vi "construct_response_generic.vi"(0 "command in":T3=enum."configure_rf", 1 "Status":T2, 5 "generic_info":string, 7 "datatype":T1, 9 "data in":variant, 11 "error in (no error) 2":errorcluster, 12 "source":string) -> (6 "Multipart message":string[](array[string]), 8 "Multipart message DVR out":refnum<data-value>, 14 "parameters JSON":string, 15 "error out 2":errorcluster)   [LabVIEW 2019, in "mmW_commands.lvlib"]
uses:
  mmW_commands.lvlib
  TypeDefs/commands.ctl
  TypeDefs/response status.ctl
  typedefs/datatypes_.ctl
  typedefs/Response_paramaters.ctl
  <vilib>/addons/_JKI.lib/Serialization/JSON/JKI JSON Serialization.lvlib
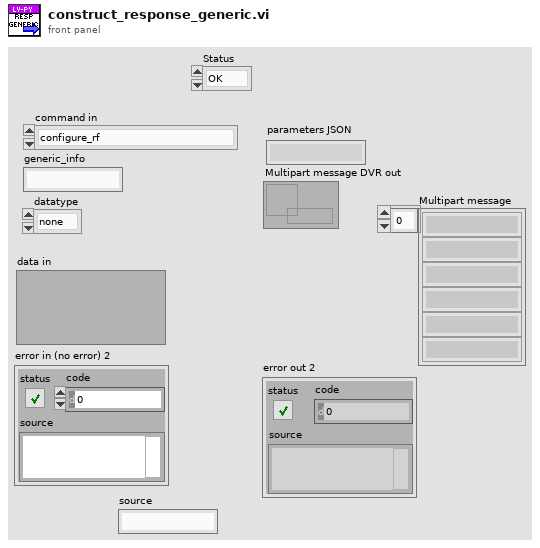
[diagram p1: front panel]
types:
  T1 = typedef "mmW_commands.lvlib/datatypes_.ctl" = enum16{"none", "string", "interleaved_I16", "interleaved_I32", "I16_array", "I32_array", "JSONstring"}
  T2 = typedef "mmW_commands.lvlib/response status.ctl" = enum16{"OK", "Error", "Warning", "Unknown"}
  T3 = typedef "mmW_commands.lvlib/commands.ctl" = enum16{"configure_fs", "configure_rf", "configure_trigger", "equalization_enable", "equalization_start", "lo_sync_enable", "equalization_stop", "get_instrument_status", "get_versions", "initialize_hw", "pop_rx", "set_log_level", "Shutdown", "start", "start_instrument_app", "stop", "trans", "transceive", "trigger_burst", "trigger_sync_enable", "Write TX", "resp_generic", "resp_waveform", "send_trigger", "fetch", "transceive2"}
  T4 = typedef "mmW_commands.lvlib/Response_paramaters.ctl" = cluster{"generic_info":string, "datatype":string, "source":string}
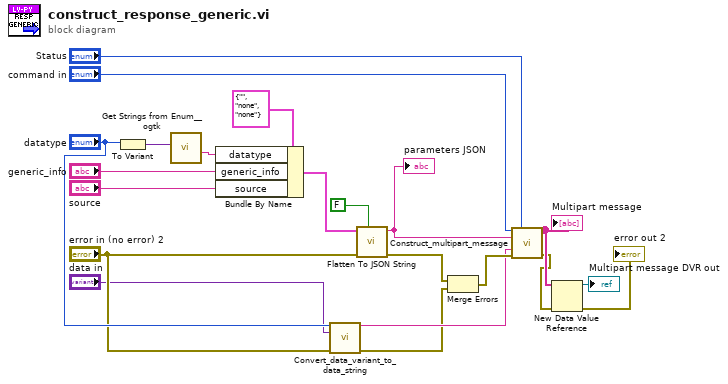
[diagram p0: block diagram]
diagram:
  n1 = To Variant(anything="datatype") -> (Variant=w14:variant)
  n2 = call <userlib>:"Get Strings from Enum__ogtk.vi"("Enum"=w14) -> ("String Value"=w13:string)  [unwired: 7 in, 3 out]
  n3 = Bundle By Name(cluster=T4 {"generic_info"="", "datatype"="none", "source"="none"} ("response data"), "datatype"=w13, "generic_info"="generic_info", "source"="source") -> (w20:T4)
  n4 = call "Convert_data_variant_to_data_string.vi"("datatype"="datatype", "data in"="data in", "error in (no error)"="error in (no error) 2") -> ("String"=w6:string, "error out"=w5:errorcluster)  [unwired: 11 in]
  n5 = call <vilib>:"Flatten To JSON String.vi"("Multiline (T)"=FALSE, "error in (no error)"="error in (no error) 2", "Variant"=w20) -> ("error out"=w12:errorcluster, "JSON String"=w17:string)  [unwired: 7 in]
  "parameters JSON" <- w17
  n6 = Merge Errors(w12, w5) -> (w11:errorcluster)
  n7 = call "Construct_multipart_message.vi"("command"="command in", "Status"="Status", "parameters (JSON)"=w17, "data in"=w6, "error in (no error)"=w11) -> ("Multipart message"=w4:string[], "error out"=w2:errorcluster)  [unwired: 7 in, 2 out]
  "Multipart message" <- w4
  n8 = New Data Value Reference(data value=w4, error in=w2) -> (data value reference=→"Multipart message DVR out":refnum<data-value>, error out=→"error out 2":errorcluster)
